vi "ManualControlL0SumnAddNOGENASICTEST.vi"(11 "Instrument VISA in":T1={"AWG VISA"="AgilentGenerator1", "Oscilloscope  VISA "="AgilentOsciloscope", "Integration Board IP"="172.16.17.47", "connection ID"=refnum, "report out"=refnum, "report file path"=path "C:/Documents and Settings/CTA_LAB01/Desktop/L0_Asic/L0 Asic Test Data"}) -> (0 "error out":errorcluster, 3 "Instrument VISA out":T1={"AWG VISA"="AgilentGenerator1", "Oscilloscope  VISA "="AgilentOsciloscope", "Integration Board IP"="172.16.7.43", "connection ID"=refnum, "report out"=refnum, "report file path"=path "C:/Documents and Settings/CTA_LAB01/Desktop/L0_Asic/L0 Asic Test Data"})   [LabVIEW 2012]
uses:
  <vilib>/Utility/NIReport.llb/NI_report.lvclass
  <vilib>/Utility/NIReport.llb/HTML/NI_HTML.lvclass
panel:
  out "element":i32=127
  in  "index":i32
  in  "Channels \nCombinations":i32[](array[numeric])=[3, 12, 48, 96, 7, 28, 112, 15, 120, 31, 124, 63, 126, 127]
  in  "error in (no error)":errorcluster
  in  "stop":bool
  in  "Enable 6":bool=TRUE
  in  "Enable 4":bool=TRUE
  in  "Enable 5":bool=TRUE
  in  "Enable 2":bool=TRUE
  in  "Enable 3":bool=TRUE
  in  "Enable 0":bool=TRUE
  in  "Enable 1":bool=TRUE
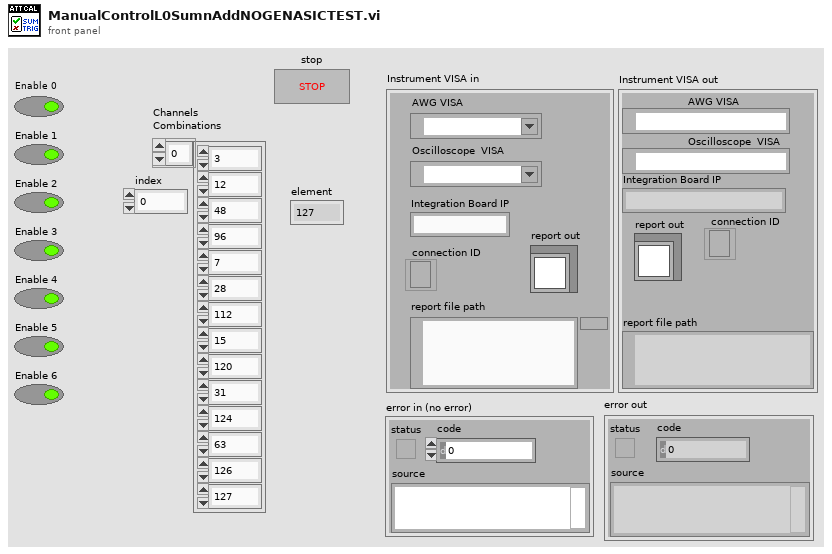
[diagram p1: front panel]
types:
  T1 = cluster{"AWG VISA":refnum<visa-resource-name>, "Oscilloscope  VISA ":refnum<visa-resource-name>, "Integration Board IP":string, "connection ID":refnum<k5>, "report out":refnum<class "NI_report.lvclass">, "report file path":path}
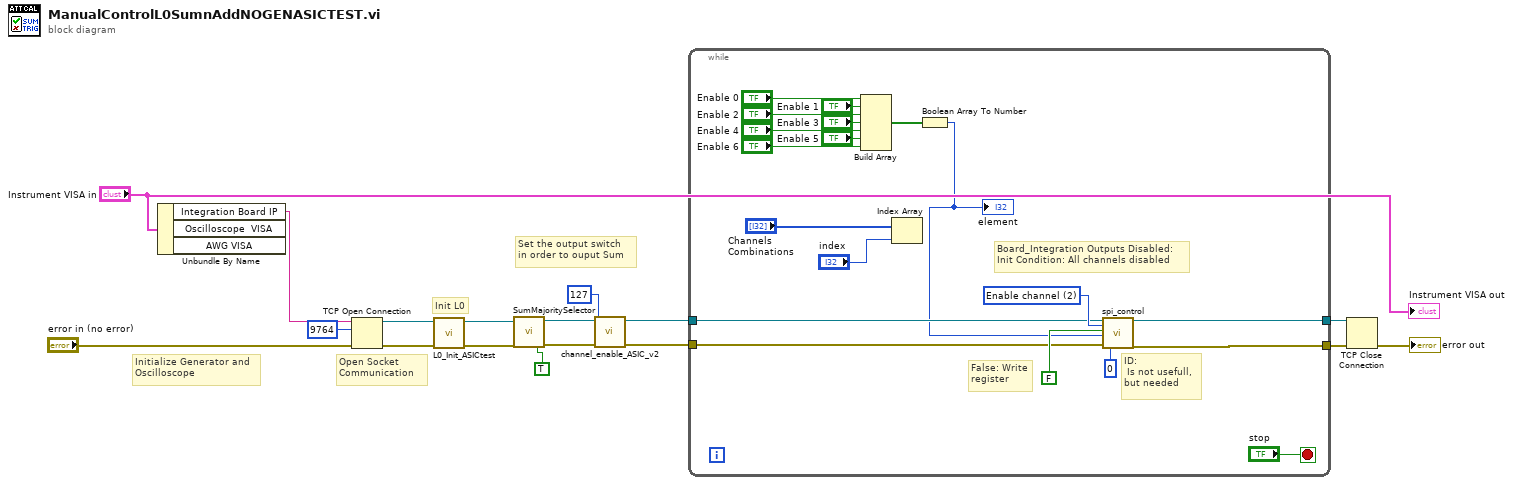
[diagram p0: block diagram]
diagram:
  # "Initialize Generator and \nOscilloscope"
  # "Init L0"
  # "Set the output switch\nin order to ouput Sum"
  # "Open Socket\nCommunication"
  n1 = Unbundle By Name("Instrument VISA in") -> ("Integration Board IP"=w15:string)  [unwired: 2 out]
  n2 = TCP Open Connection(address=w15, remote port or service name=u16 9764, error in (no error)="error in (no error)") -> (connection ID=w13:refnum<k5>, error out=w12:errorcluster)  [unwired: 2 in]
  n3 = call "L0_Init_ASICtest.vi"("error in"=w12, "connection ID in"=w13) -> ("error out"=w10:errorcluster, "connection ID out"=w11:refnum<k5>)  [unwired: 8 in]
  n4 = call "SumMajoritySelector.vi"("On Sum\nOff Majority"=TRUE ("On Sum\nOff Majority"), "error in (no error)"=w10, "connection ID"=w11) -> ("error out"=w4:errorcluster, "connection ID out"=w2:refnum<k5>)  [unwired: 5 in]
  n5 = call "channel_enable_ASIC_v2.vi"("error in"=w4, "Channel Combination"=u32 127, "Connection ID in"=w2) -> ("error out"=w3:errorcluster, "Connection ID out"=w1:refnum<k5>)  [unwired: 7 in]
  n6 = while {
    tunnel: w1 -> [w23]
    tunnel: w3 -> [w24]
    tunnel: [w21] -> w7
    tunnel: [w22] -> w8
    stop <- "stop" stop-if-true
    w35 = u16 2 items=["Attenuation", "Clipping", "Enable channel", "Delay line", "ASIC"] ("Device")
    # "False: Write\nregister"
    # "ID:\n Is not usefull, \nbut needed"
    # "Board_Integration Outputs Disabled:\nInit Condition: All channels disabled"
    n7 = Build Array("Enable 0", "Enable 1", "Enable 2", "Enable 3", "Enable 4", "Enable 5", "Enable 6") -> (w33:bool[])
    n8 = Index Array(array="Channels \nCombinations", index="index") -> ()  [unwired: 1 out]
    n9 = Boolean Array To Number(Boolean array=w33) -> (number=w18:u32)
    "element" <- w18
    n10 = call "spi_control.vi"("connection ID"=w23, "Device"=w35, "Read/#write"=FALSE, "Data"=w18, "error out 3"=w24, "Id in"=0) -> ("connection ID out"=w22:refnum<k5>, "error out 2"=w21:errorcluster)  [unwired: 6 in, 6 out]
  }
  n11 = TCP Close Connection(connection ID=w8, error in (no error)=w7) -> (error out=→"error out":errorcluster)  [unwired: 1 in, 1 out]
  "Instrument VISA out" <- "Instrument VISA in"
